vi "FPGA Main.vi"() -> ()   [LabVIEW 2016]
uses:
  Type Def Ctrls/FPGA ctrls/FPGA State.ctl
  Type Def Ctrls/FPGA ctrls/Input Channels.ctl
  Type Def Ctrls/FPGA ctrls/Output Channels.ctl
  Type Def Ctrls/FPGA ctrls/Manual Setpoint.ctl
  Type Def Ctrls/FPGA ctrls/PID output selection.ctl
  Type Def Ctrls/FPGA ctrls/Reset PID.ctl
  <vilib>/rvi/Analysis/control/PID/Typedef/niFpgaPID_PIDGains.ctl
  <vilib>/rvi/Analysis/control/PID/Typedef/niFpgaPID_OutputRange.ctl
  Type Def Ctrls/FPGA ctrls/PID status.ctl
  <vilib>/LabVIEW Targets/FPGA/cRIO/shared/nicrio_ModuleControls/nicrio_cRIO-9219_ConversionTime.ctl
  Type Def Ctrls/FPGA ctrls/NI9219VoltageRange.ctl
  Type Def Ctrls/FPGA ctrls/fast output sampling rate.ctl
  Type Def Ctrls/FPGA ctrls/underflow warning level.ctl
  <vilib>/rvi/Emulation/niFpgaSctlEmulationGetInTimedLoop.vi
  <vilib>/rvi/Emulation/niFpgaProcessEmulError.vi
  <vilib>/rvi/Emulation/niFpgaGetClockAttributes.vi
  <vilib>/rvi/Emulation/niFpgaEmulationReportErrorSimple.vi
  <vilib>/rvi/eio/common/nirviEmuTemplateMethod_errors.vi
  <vilib>/rvi/Emulation/niFpgaCriticalErrorInLSC.vi
  <vilib>/rvi/eio/common/nirviEmuTemplatePropertySet_noerrors.vi
  <vilib>/eio/EIONode/EIONode.xnode
  <vilib>/eio/EIOPropertyNode/EIOPropertyNode.xnode
  <vilib>/LabVIEW Targets/FPGA/cRIO/shared/nicrio_ModuleControls/nicrio_cRIO-9219_VoltageRange.ctl
  <vilib>/rvi/eio/common/nirviEmuTemplatePropertyGet_errors.vi
  <vilib>/rvi/eio/common/nirviEmuTemplatePropertyGet_noerrors.vi
  <vilib>/rvi/eio/common/nirviEmuTemplatePropertySet_errors.vi
panel:
  out "IRQ counts":u64
  out "time stamp (ms)":u64
  out "temperature channel":i16
  out "Chassis Temperature":sgl
  in  "PID output channel":T1
  in  "Enable Watchdog":bool
  in  "Pet Watchdog":bool
  in  "Watchdog Timeout Period (ticks)":u64=200000000 format="%.0p"
  out "Watchdog Timed Out?":bool=TRUE
  out "Time Since Last Pet":u64
  in  "flush queue?":bool
  in  "underflow warning level":T2
  in  "Update \n9219 settings":bool
  in  "fast output sampling rate":T3=100000 min=1 max=100000
  out "Fast output queue idle?":bool
  in  "9269 Fast Output Enabled":bool
  out "ticks":i64
  in  "RTMain Running?":bool
  out "CJC R_T":sgl
  in  "Input voltage range":T4[](array[typedef])=[0, 0, 0, 0] items=["+/- 60V", "+/- 15V", "+/- 4V", "+/- 1V", "+/- 125mV"]
  in  "9219 Conversion Time":T5
  out "PID status":T6
  in  "PID output ranges":T7={"output high (Inf)"=10.0, "output low (-Inf)"=-10.0} {"output low (-Inf)" min=-10 max=10; "output high (Inf)" min=0 max=10}
  in  "PID gains":T8 {"filter coefficient" min=0 max=1; "proportional gain" step=0.125}
  out "Output Channel values":T9
  in  "reset PID?":T10
  in  "PID input channel":T1
  in  "Setpoint for \nPID input chn":T11
  in  "Set output":T9=[0.0, 0.0, 0.0, 0.0]
  out "Input Channel values":T12 format="%#10_8p"
  in  "FPGA state":T13
  in  "Relay Switch Matrix":u32 format="%08x"
  # "Created by Quan Qing, QingLAB @ ASU. \nhttps://qinglab.physics.asu.edu"
  # "General Settings"
  # "Remote Inputs"
  # "Fast output settings"
  # "I/O records"
  # "PID settings"
  # "WatchDog Settings"
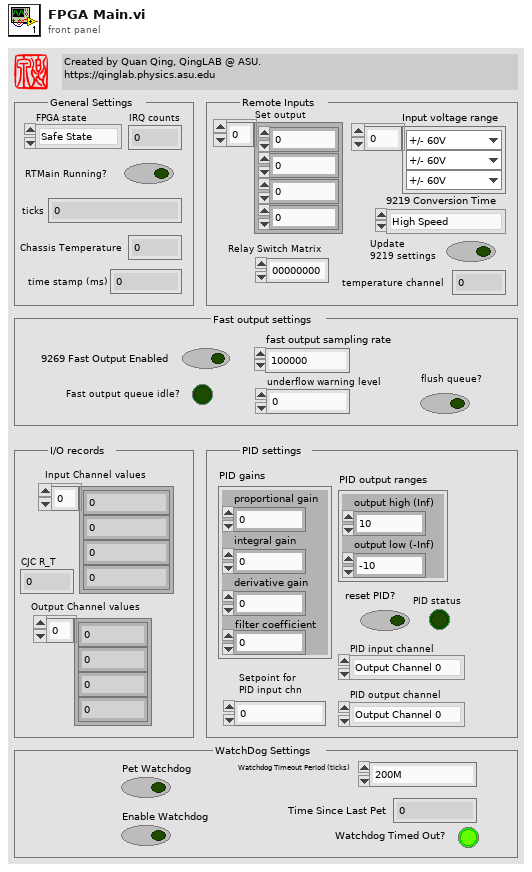
[diagram p1: front panel]
types:
  T1 = typedef "PID output selection.ctl" = enum16{"Output Channel 0", "Output Channel 1", "Output Channel 2", "Output Channel 3", "PID Disabled"}
  T2 = typedef "underflow warning level.ctl" = u32
  T3 = typedef "fast output sampling rate.ctl" = u32
  T4 = typedef "NI9219VoltageRange.ctl" = u8
  T5 = typedef "nicrio_cRIO-9219_ConversionTime.ctl" = enum8{"High Speed", "Best 60 Hz Rejection", "Best 50 Hz Rejection", "High Resolution"}
  T6 = typedef "PID status.ctl" = bool
  T7 = typedef "niFpgaPID_OutputRange.ctl" = cluster{"output high (Inf)":sgl, "output low (-Inf)":sgl}
  T8 = typedef "niFpgaPID_PIDGains.ctl" = cluster{"proportional gain":sgl, "integral gain":sgl, "derivative gain":sgl, "filter coefficient":sgl}
  T9 = typedef "Output Channels.ctl" = sgl[]
  T10 = typedef "Reset PID.ctl" = bool
  T11 = typedef "Manual Setpoint.ctl" = sgl
  T12 = typedef "Input Channels.ctl" = sgl[]
  T13 = typedef "FPGA State.ctl" = enum16{"Safe State", "I/O with PID Control", "Fast Output Only"}
  T14 = cluster{"[0]":fxp<+/-,20,5>, "[1]":fxp<+/-,20,5>, "[2]":fxp<+/-,20,5>, "[3]":fxp<+/-,20,5>}
  T15 = cluster{"Input voltage range[0]":T4, "Input voltage range[1]":T4, "Input voltage range[2]":T4, "Input voltage range[3]":T4, "Input voltage range[4]":T4, "Input voltage range[5]":T4, "Input voltage range[6]":T4, "Input voltage range[7]":T4, "Input voltage range[8]":T4}
  T16 = typedef "AO channel cluster.ctl" = cluster{"AO CH 0":fxp<+/-,20,5>, "AO CH 1":fxp<+/-,20,5>, "AO CH 2":fxp<+/-,20,5>, "AO CH 3":fxp<+/-,20,5>}
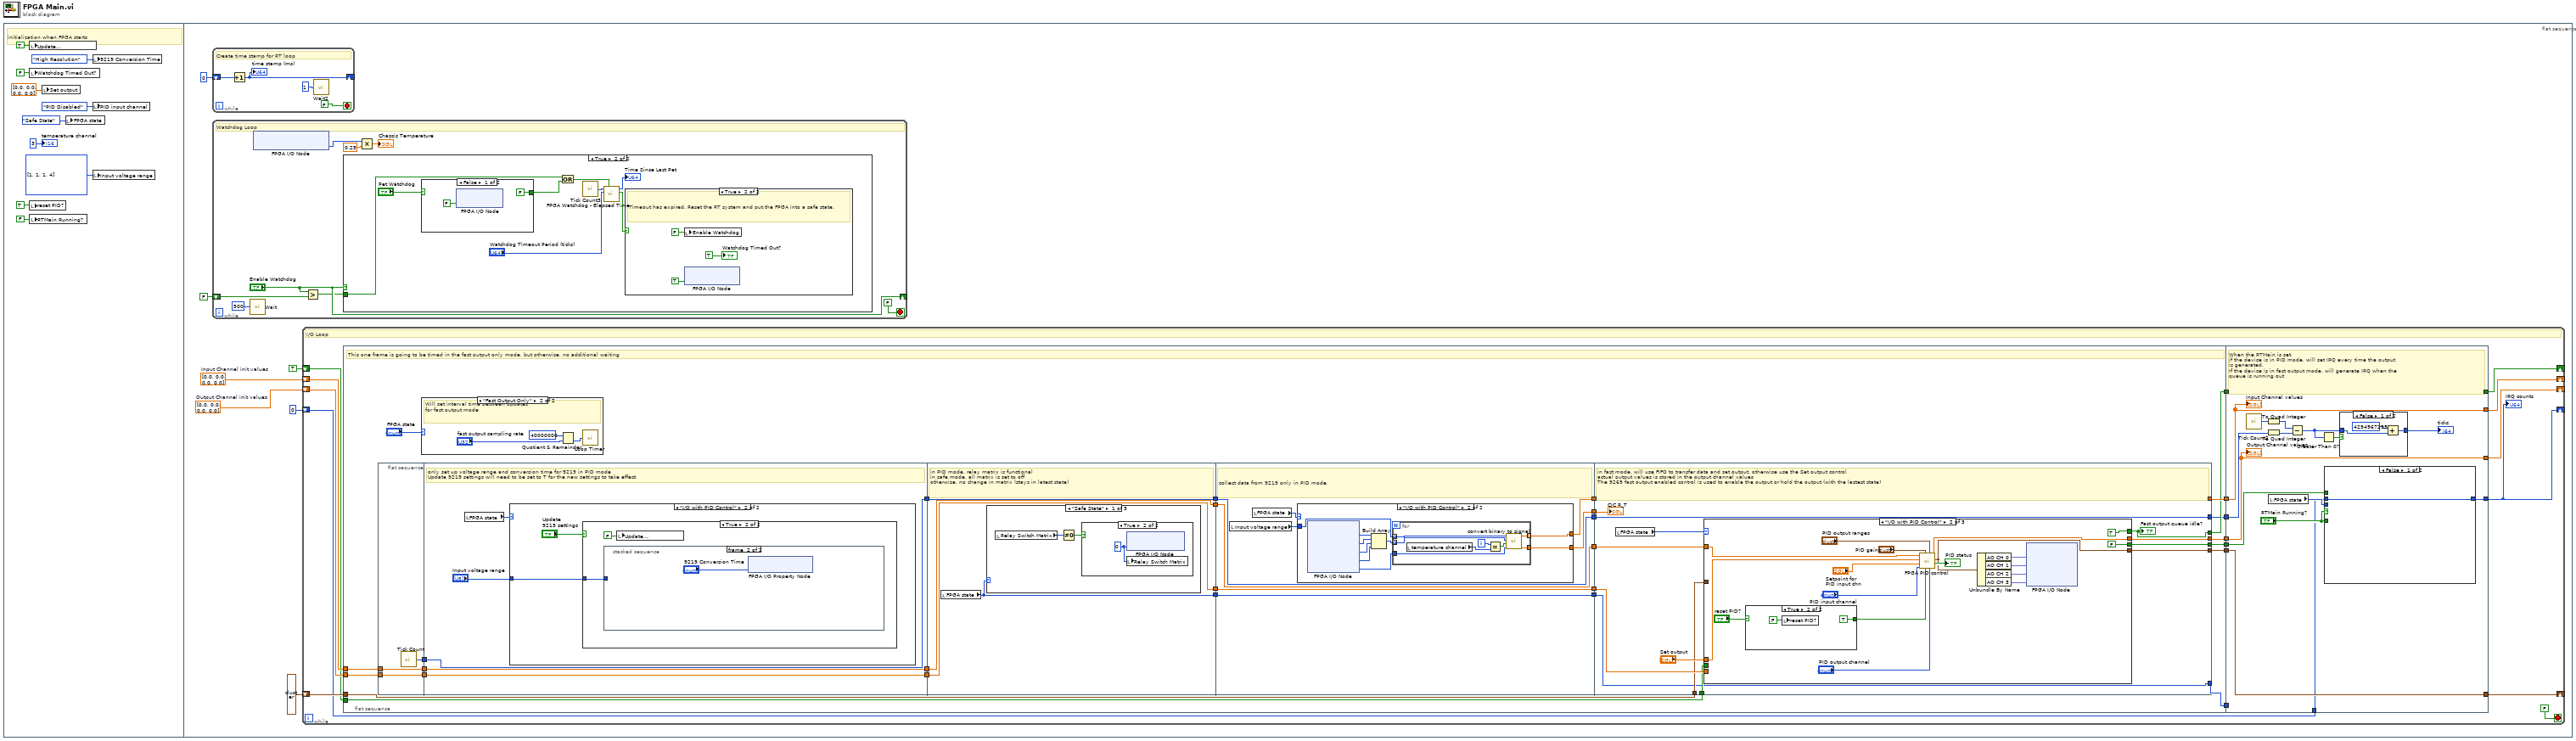
[diagram p0: block diagram]
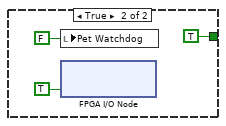
[diagram p3: hidden frame]
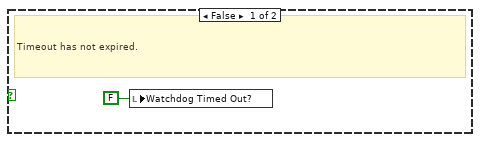
[diagram p4: hidden frame]
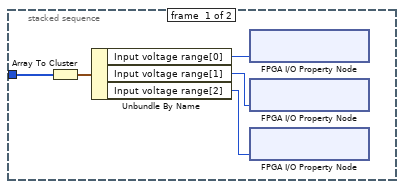
[diagram p8: hidden frame]
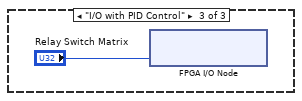
[diagram p11: hidden frame]
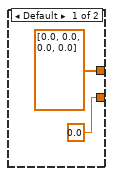
[diagram p12: hidden frame]
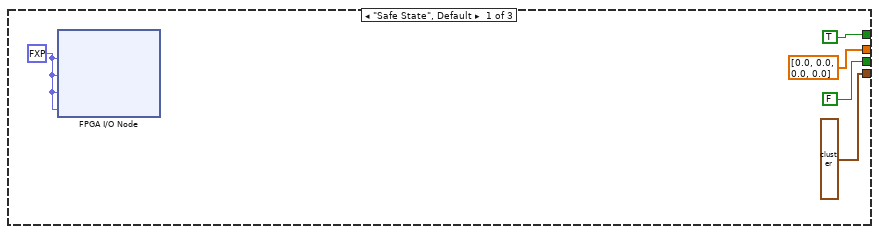
[diagram p13: hidden frame]
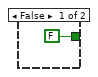
[diagram p14: hidden frame]
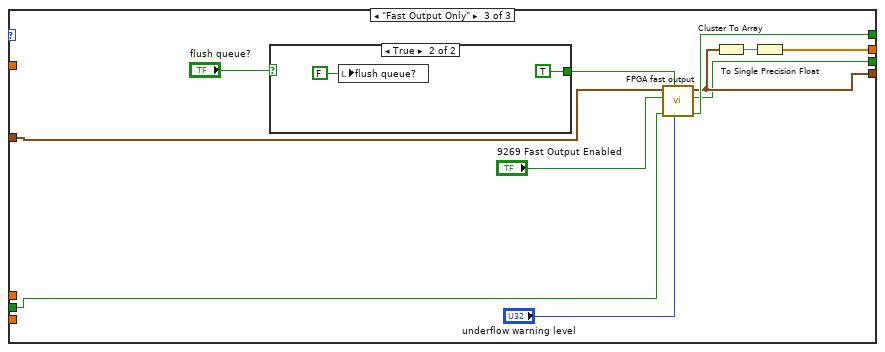
[diagram p15: hidden frame]
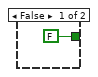
[diagram p16: hidden frame]
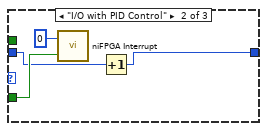
[diagram p18: hidden frame]
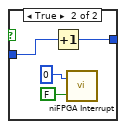
[diagram p20: hidden frame]
diagram:
  n1 = flat-sequence {
    frame #0 {
      w6 = T4[] [1, 1, 1, 4] items=["+/- 60V", "+/- 15V", "+/- 4V", "+/- 1V", "+/- 125mV"] ("Input voltage range")
      # "initialization when FPGA starts"
      n2 = local write "Update \n9219 settings"(TRUE ("Update 9219 settings")) -> ()
      n3 = local write "Watchdog Timed Out?"(FALSE ("Watchdog Timed Out?")) -> ()
      n4 = local write "reset PID?"(T10 TRUE ("reset PID?")) -> ()
      n5 = local write "RTMain Running?"(FALSE ("RTMain Running?")) -> ()
      n6 = local write "Set output"(T9 [0.0, 0.0, 0.0, 0.0] ("Set output")) -> ()
      n7 = local write "FPGA state"(FPGA_State."Safe State" ("FPGA state")) -> ()
      n8 = local write "9219 Conversion Time"(nicrio_cRIO-9219_ConversionTime."High Resolution" ("9219 Conversion Time")) -> ()
      n9 = local write "PID input channel"(PID_output_selection."PID Disabled" ("PID process channel")) -> ()
      n10 = local write "Input voltage range"(w6) -> ()
      "temperature channel" <- i16 3 ("temperature channel")
    }
    frame #1 {
      w14 = T12 [0.0, 0.0, 0.0, 0.0]  # Input Channel init values
      w13 = T9 [0.0, 0.0, 0.0, 0.0]  # Output Channel init values
      n11 = while {
        shift-right: [w20] -> _
        shift-left: u64 0 -> [w21]
        stop <- FALSE stop-if-true
        # "Create time stamp for RT loop"
        n12 = Increment(x=w21) -> (x+1=w20:u64)
        "time stamp (ms)" <- w20
        n13 = call "Wait2"("Count(mSec)"=u32 1) -> ()  [unwired: 1 out]
      }
      n14 = while "RT Watchdog Loop" {
        shift-right: ["Enable Watchdog"] -> _
        shift-left: FALSE ("Enable RT Watchdog") -> [w29]
        stop <- FALSE stop-if-true
        # "Watchdog Loop"
        n15 = call "Wait"("Count(mSec)"=u32 500) -> ()  [unwired: 1 out]
        n16 = xnode "FPGA I/O Node"() -> ("Chassis Temperature"=w24:i16)  [unwired: 1 in, 1 out]
        n17 = Greater?(x="Enable Watchdog", y=w29) -> (0:w26:bool)
        n18 = case shown="True" "Enable Watchdog" {
          tunnel: w26 -> [_ w37]
          frame False {
            # "This loop has to be explicitly enabled from the RT Main VI.  This reduces the possiblity of an endless reboot cycle."
          }
          frame True {
            n19 = case shown="False" "Pet Watchdog" {
              tunnel: [FALSE TRUE] -> w30
              frame False {
                n20 = xnode "FPGA I/O Node"("FPGA LED"=FALSE) -> ()  [unwired: 1 in, 1 out]
              }
              frame True {
                n21 = local write "Pet Watchdog"(FALSE ("Pet Watchdog")) -> ()
                n22 = xnode "FPGA I/O Node"("FPGA LED"=TRUE) -> ()  [unwired: 1 in, 1 out]
              }
            }
            n23 = Or(x=w37, y=w30) -> (x .or. y?=w36:bool)
            n24 = call "Tick Count3"() -> ("Tick Count(Ticks)"=w35:u32)
            n25 = call "FPGA Watchdog - Elapsed Time.vi"("Reset"=w36, "Timeout Period"="Watchdog Timeout Period (ticks)", "Current Time"=w35) -> ("Timeout"=w32:bool, "Elapsed Time"=→"Time Since Last Pet":u64)  [unwired: 7 in]
            n26 = case shown="True" w32 {
              frame False {
                # "Timeout has not expired."
                n27 = local write "Watchdog Timed Out?"(FALSE ("Watchdog Timed Out?")) -> ()
              }
              frame True {
                # "Timeout has expired. Reset the RT system and put the FPGA into a safe state."
                n28 = local write "Enable Watchdog"(FALSE ("Enable RT Watchdog")) -> ()
                n29 = xnode "FPGA I/O Node"("System Reset"=TRUE ("RT Reset on Watchdog Failure?")) -> ()  [unwired: 1 in, 1 out]
                "Watchdog Timed Out?" <- TRUE ("Watchdog Timed Out?")
              }
            }
          }
        }
        n30 = Multiply(x=w24, y=sgl 0.25) -> (x*y=→"Chassis Temperature":sgl)
      }
      n31 = while "I/O loop" {
        shift-right: [w60] -> _
        shift-left: w13 -> [w63]
        shift-right: [w62] -> _
        shift-left: w14 -> [w61]
        shift-right: [w59] -> _
        shift-left: T14 {"[0]"=0.0, "[1]"=0.0, "[2]"=0.0, "[3]"=0.0} ("fast output out") -> [w58]
        shift-right: [w57] -> _
        shift-left: TRUE ("fast queue idle out") -> [w56]
        shift-right: [w47] -> _
        shift-left: u64 0 -> [w48]
        stop <- FALSE stop-if-true
        # "I/O Loop"
        n32 = flat-sequence {
          tunnel: w63 -> [w76]
          tunnel: w61 -> [w74]
          tunnel: w58 -> [w71]
          tunnel: w56 -> [w69]
          tunnel: [w75] -> w55
          tunnel: [w73] -> w54
          tunnel: [w72] -> w53
          tunnel: [w70] -> w52
          tunnel: [w67] -> w51
          tunnel: [w66] -> w50
          tunnel: [w65] -> w49
          tunnel: [w217] -> w57
          tunnel: [w218] -> w59
          tunnel: [w205] -> w60
          tunnel: [w206] -> w62
          tunnel: w55 -> [w206]
          tunnel: w54 -> [w205]
          tunnel: w53 -> [w218]
          tunnel: w52 -> [w217]
          tunnel: w51 -> [w210]
          tunnel: w50 -> [_]
          tunnel: w49 -> [w208]
          tunnel: [w204] -> w47
          tunnel: w48 -> [w203]
          frame #0 {
            # "This one frame is going to be timed in the fast output only mode, but otherwise, no additional waiting"
            n33 = flat-sequence {
              tunnel: w74 -> [w97]
              tunnel: w76 -> [w98]
              tunnel: [w98] -> w92
              tunnel: [w97] -> w91
              tunnel: [w96] -> w90
              tunnel: [w103] -> w89
              tunnel: [w102] -> w88
              tunnel: w92 -> [w103]
              tunnel: w91 -> [w102]
              tunnel: [w101] -> w87
              tunnel: w90 -> [w101]
              tunnel: [w114] -> w86
              tunnel: [w117] -> w85
              tunnel: [w116] -> w84
              tunnel: w89 -> [w117]
              tunnel: w88 -> [w116]
              tunnel: [w115] -> w83
              tunnel: w87 -> [w115]
              tunnel: [w127] -> w82
              tunnel: [w129] -> w81
              tunnel: [w128] -> w80
              tunnel: w86 -> [w127]
              tunnel: w85 -> [w129]
              tunnel: w84 -> [w128]
              tunnel: [w126] -> w79
              tunnel: w83 -> [w126]
              tunnel: [w125] -> w78
              tunnel: [w124] -> w77
              tunnel: w82 -> [w151]
              tunnel: w81 -> [w161]
              tunnel: w80 -> [w160]
              tunnel: w79 -> [w152]
              tunnel: w78 -> [w159]
              tunnel: w77 -> [w158]
              tunnel: w71 -> [w156]
              tunnel: [w155] -> w70
              tunnel: w69 -> [w154]
              tunnel: [w159] -> w75
              tunnel: [w153] -> w73
              tunnel: [w157] -> w72
              tunnel: [w152] -> w67
              tunnel: [w151] -> w66
              tunnel: [w150] -> w65
              frame #0 {
                n34 = call "Tick Count"() -> ("Tick Count(Ticks)"=w96:u32)
              }
              frame #1 {
                # "only set up voltage range and conversion time for 9219 in PID mode\nUpdate 9219 settings will need to be set to T for the new settings to take effect"
                n35 = local read "FPGA state"() -> (w99:T13)
                n36 = case shown="\"I/O with PID Control\"" w99 {
                  tunnel: "Input voltage range" -> [_ w105]
                  frame Default {
                  }
                  frame "I/O with PID Control" {
                    n37 = case shown="True" "Update \n9219 settings" {
                      tunnel: w105 -> [_ w107]
                      frame False {
                      }
                      frame True {
                        n38 = stacked-sequence {
                          tunnel: w107 -> [w111 _]
                          frame #0 {
                            n39 = Array To Cluster(array=w111) -> (cluster=w112:T15)
                            n40 = Unbundle By Name(w112) -> ("Input voltage range[0]"=w110:T4, "Input voltage range[1]"=w109:T4, "Input voltage range[2]"=w108:T4)
                            n41 = xnode "FPGA I/O Property Node"("Voltage Range"=w110) -> ()  [unwired: 1 in, 1 out]
                            n42 = xnode "FPGA I/O Property Node"("Voltage Range"=w109) -> ()  [unwired: 1 in, 1 out]
                            n43 = xnode "FPGA I/O Property Node"("Voltage Range"=w108) -> ()  [unwired: 1 in, 1 out]
                          }
                          frame #1 {
                            n44 = xnode "FPGA I/O Property Node"("Conversion Time"="9219 Conversion Time") -> ()  [unwired: 1 in, 1 out]
                          }
                        }
                        n45 = local write "Update \n9219 settings"(FALSE ("Update 9219 settings")) -> ()
                      }
                    }
                  }
                }
              }
              frame #2 {
                # "in PID mode, relay matrix is functional\nin safe mode, all matrix is set to off\notherwise, no change in matrix (stays in latest state)"
                n46 = local read "FPGA state"() -> (w114:T13)
                n47 = case shown="\"Safe State\"" w114 {
                  frame "Safe State" {
                    n48 = local read "Relay Switch Matrix"() -> (w119:u32)
                    n49 = Not Equal To 0?(x=w119) -> (x != 0?=w118:bool)
                    n50 = case shown="True" w118 {
                      frame False {
                      }
                      frame True {
                        w120 = u32 0 ("Mod2/DO31:0")
                        n51 = xnode "FPGA I/O Node"("Mod2/DO31:0"=w120) -> ()  [unwired: 1 in, 1 out]
                        n52 = local write "Relay Switch Matrix"(w120) -> ()
                      }
                    }
                  }
                  frame "Fast Output Only" {
                  }
                  frame "I/O with PID Control" {
                    n53 = xnode "FPGA I/O Node"("Mod2/DO31:0"="Relay Switch Matrix") -> ()  [unwired: 1 in, 1 out]
                  }
                }
              }
              frame #3 {
                # "collect data from 9219 only in PID mode"
                n54 = local read "Input voltage range"() -> (w122:T4[])
                n55 = local read "FPGA state"() -> (w123:T13)
                n56 = case shown="\"I/O with PID Control\"" w123 {
                  tunnel: w122 -> [_ w135]
                  tunnel: [sgl[] [0.0, 0.0, 0.0, 0.0] ("signal") w133] -> w125
                  tunnel: [sgl 0.0 ("R_T") w132] -> w124
                  frame Default {
                  }
                  frame "I/O with PID Control" {
                    n57 = xnode "FPGA I/O Node"() -> ("Mod3/CH0"=w140:i32, "Mod3/CH1"=w139:i32, "Mod3/CH2"=w138:i32, "Mod3/CH3"=w137:i32, "Mod3/CJC3"=w134:u32)  [unwired: 5 in, 5 out]
                    n58 = Build Array(w140, w139, w138, w137) -> (w136:i32[])
                    n59 = for {
                      tunnel: [w148] -> w133 mode=indexing
                      tunnel: w136 -> [w147] mode=indexing
                      tunnel: w135 -> [w146] mode=indexing
                      tunnel: w134 -> [w145]
                      tunnel: [w144] -> w132
                      i -> [w143]
                      n60 = local read "temperature channel"() -> (w141:i16)
                      n61 = Equal?(x=w143, y=w141) -> (x = y?=w142:bool)
                      n62 = call "convert binary to signal.vi"("Binary CJC"=w145, "Thermocouple data?"=w142, "Binary raw"=w147, "Voltage Range"=w146) -> ("R_T"=w144:sgl, "signal"=w148:sgl)  [unwired: 6 in]
                    }
                  }
                }
              }
              frame #4 {
                # "in fast mode, will use FIFO to transfer data and set output. otherwise use the Set output control\nactual output values is stored in the output channel values\nThe 9269 fast output enabled control is used to enable the output or hold the output (with the lastest state)"
                n63 = local read "FPGA state"() -> (w149:T13)
                n64 = case shown="\"I/O with PID Control\"" w149 {
                  tunnel: w160 -> [_ w183 _]
                  tunnel: "Set output" -> [_ w184 _]
                  tunnel: w161 -> [_ _ _]
                  tunnel: [T9 [0.0, 0.0, 0.0, 0.0] ("Output Channels shadow") w178 w193] -> w153
                  tunnel: [T14 {"[0]"=0.0, "[1]"=0.0, "[2]"=0.0, "[3]"=0.0} ("fast output out") w173 w195] -> w157
                  tunnel: w156 -> [_ _ w199]
                  tunnel: w154 -> [_ _ w197]
                  tunnel: [TRUE ("fast queue idle out") TRUE ("fast queue idle out") w196] -> w155
                  tunnel: [FALSE ("underflow warning") FALSE ("underflow warning") w191] -> w150
                  frame "Safe State", Default {
                    w166 = fxp<+/-,20,5> 0.0 ("Mod1/AO0")
                    n65 = xnode "FPGA I/O Node"("Mod1/AO0"=w166, "Mod1/AO1"=w166, "Mod1/AO2"=w166, "Mod1/AO3"=w166) -> ()  [unwired: 4 in, 4 out]
                  }
                  frame "I/O with PID Control" {
                    n66 = case shown="True" "reset PID?" {
                      tunnel: [FALSE TRUE] -> w170
                      frame False {
                      }
                      frame True {
                        n67 = local write "reset PID?"(T10 FALSE ("reset PID?")) -> ()
                      }
                    }
                    n68 = call "FPGA PID control.vi"("PID output channel"="PID output channel", "output ranges"="PID output ranges", "reset pid"=w170, "PID gains"="PID gains", "PID input channel"="PID input channel", "setpoint"="Setpoint for \nPID input chn", "set output"=w184, "inputs"=w183) -> ("PID status"=→"PID status":T6, "to AO channels"=w173:T16, "actual outputs"=w178:sgl[])  [unwired: 1 in]
                    n69 = Unbundle By Name(w173) -> ("AO CH 0"=w177:fxp<+/-,20,5>, "AO CH 1"=w176:fxp<+/-,20,5>, "AO CH 2"=w175:fxp<+/-,20,5>, "AO CH 3"=w174:fxp<+/-,20,5>)
                    n70 = xnode "FPGA I/O Node"("Mod1/AO0"=w177, "Mod1/AO1"=w176, "Mod1/AO2"=w175, "Mod1/AO3"=w174) -> ()  [unwired: 4 in, 4 out]
                  }
                  frame "Fast Output Only" {
                    n71 = case shown="True" "flush queue?" {
                      tunnel: [FALSE TRUE] -> w189
                      frame False {
                      }
                      frame True {
                        n72 = local write "flush queue?"(FALSE ("flush queue?")) -> ()
                      }
                    }
                    n73 = call "FPGA fast output.vi"("underflow warning level"="underflow warning level", "flush queue?"=w189, "fast queue idle in"=w197, "9269 Output Enabled"="9269 Fast Output Enabled", "fast output in"=w199) -> ("fast queue idle out"=w196:bool, "underflow warning"=w191:bool, "fast output out"=w195:T14)  [unwired: 4 in]
                    n74 = Cluster To Array(cluster=w195) -> (array=w194:fxp<+/-,20,5>[])
                    n75 = To Single Precision Float(number=w194) -> (single precision float=w193:sgl[])
                  }
                }
                "Fast output queue idle?" <- w155
                "CJC R_T" <- w158
              }
            }
            n76 = case shown="\"Fast Output Only\"" "FPGA state" {
              frame Default {
              }
              frame "Fast Output Only" {
                # "Will set interval time between updates \nfor fast output mode"
                n77 = Quotient & Remainder(x=u32 40000000 ("y"), y="fast output sampling rate") -> (floor(x/y)=w95:T3)  [unwired: 1 out]
                n78 = call "Loop Timer"("Count(Ticks)"=w95) -> ()  [unwired: 1 out]
              }
            }
          }
          frame #1 {
            # "When the RTMain is set, \nif the device is in PID mode, will set IRQ every time the output\nis generated.\nIf the device is in fast output mode, will generate IRQ when the \nqueue is running out"
            n79 = call "Tick Count2"() -> ("Tick Count(Ticks)"=w216:u32)
            n80 = To Quad Integer(1:w216) -> (0:w215:i64)
            n81 = To Quad Integer(1:w210) -> (0:w214:i64)
            n82 = local read "FPGA state"() -> (w207:T13)
            n83 = Subtract(x=w215, y=w214) -> (x-y=w212:i64)
            n84 = Greater Than 0?(x=w212) -> (x > 0?=w213:bool)
            n85 = case shown="False" "RTMain Running?" {
              tunnel: "RTMain Running?" -> [_ w223]
              tunnel: w207 -> [_ w224]
              tunnel: w208 -> [_ w222]
              tunnel: [w219 w221] -> w204
              tunnel: w203 -> [w219 w220]
              frame False {
              }
              frame True {
                n86 = case shown="\"Safe State\", Default" w224 {
                  tunnel: w223 -> [_ w228 _]
                  tunnel: w222 -> [_ _ w232]
                  tunnel: [w225 w227 w230] -> w221
                  tunnel: w220 -> [w225 w226 w231]
                  frame "Safe State", Default {
                  }
                  frame "I/O with PID Control" {
                    n87 = call <vilib>:"niFPGA Interrupt.vi"("Wait Until Cleared (F)"=w228, "IRQ Number (0)"=u8 0 ("IRQ Bit (0-31)")) -> ()  [unwired: 1 in]
                    n88 = Increment(x=w226) -> (x+1=w227:u64)
                  }
                  frame "Fast Output Only" {
                    n89 = case shown="False" w232 {
                      tunnel: w231 -> [w233 w235]
                      tunnel: [w233 w234] -> w230
                      frame False {
                      }
                      frame True {
                        n90 = Increment(x=w235) -> (x+1=w234:u64)
                        n91 = call <vilib>:"niFPGA Interrupt.vi"("Wait Until Cleared (F)"=FALSE, "IRQ Number (0)"=u8 0 ("IRQ Bit (0-31)")) -> ()  [unwired: 1 in]
                      }
                    }
                  }
                }
              }
            }
            n92 = case shown="False" w213 {
              tunnel: w212 -> [w239 w241]
              tunnel: [w238 w241] -> w211
              frame False {
                n93 = Add(x=i64 4294967295, y=w239) -> (x+y=w238:i64)
              }
              frame True {
              }
            }
            "ticks" <- w211
            "Input Channel values" <- w206
            "Output Channel values" <- w205
          }
        }
        "IRQ counts" <- w47
      }
    }
  }
